vi "LEP_RV_OnAbort.vi"(8 "error in (no error)":errorcluster) -> (0 "error out":errorcluster)   [LabVIEW 2011]
doc: "Download and execute built VxWorks downloadable module and attach the LabVIEW Embedded debuger."
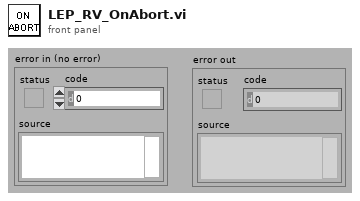
[diagram p1: front panel]
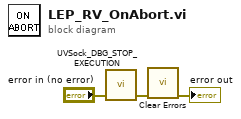
[diagram p0: block diagram]
diagram:
  n1 = call "UVSock_DBG_STOP_EXECUTION.vi"("error in (no error)"="error in (no error)") -> ("error out"=w2:errorcluster)  [unwired: 4 in]
  n2 = call <vilib>:"Clear Errors.vi"("error in (no error)"=w2) -> ("error out"=→"error out":errorcluster)  [unwired: 6 in]
